vi "serial_load.vi"(5 "new_data_available":bool, 7 "read_buffer_in":string, 8 "data_available_in":T1, 9 "freq_available_in":bool, 10 "s11_data_array_in":dbl[][](array[numeric]), 11 "freq_array_in":dbl[](array[numeric])) -> (0 "data_available_out":T1, 1 "freq_available_out":bool, 2 "data_array_out":dbl[][](array[numeric]), 3 "freq_array_out":dbl[](array[numeric]), 4 "sweep_data":dbl[](array[numeric]), 6 "sweep_data_available":bool)   [LabVIEW 2025]
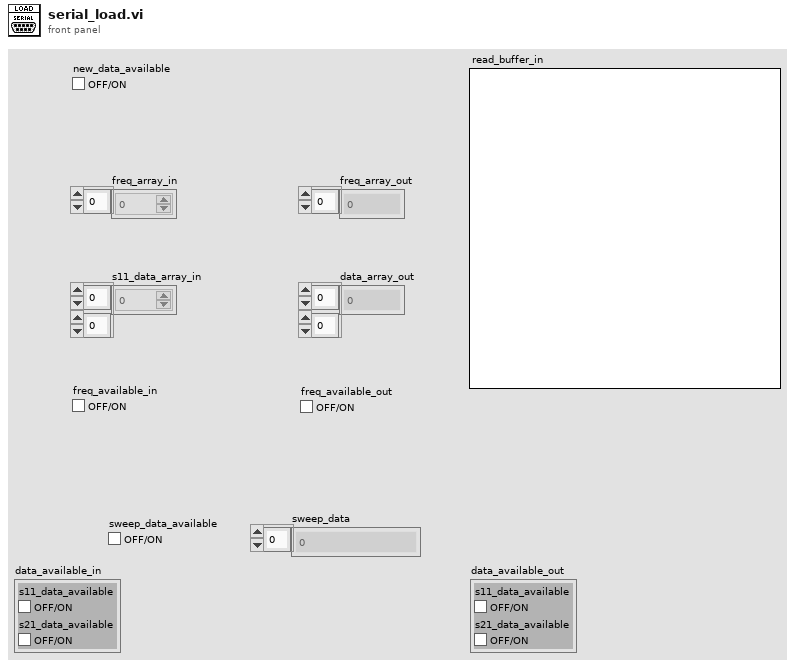
[diagram p1: front panel]
types:
  T1 = cluster{"s11_data_available":bool, "s21_data_available":bool}
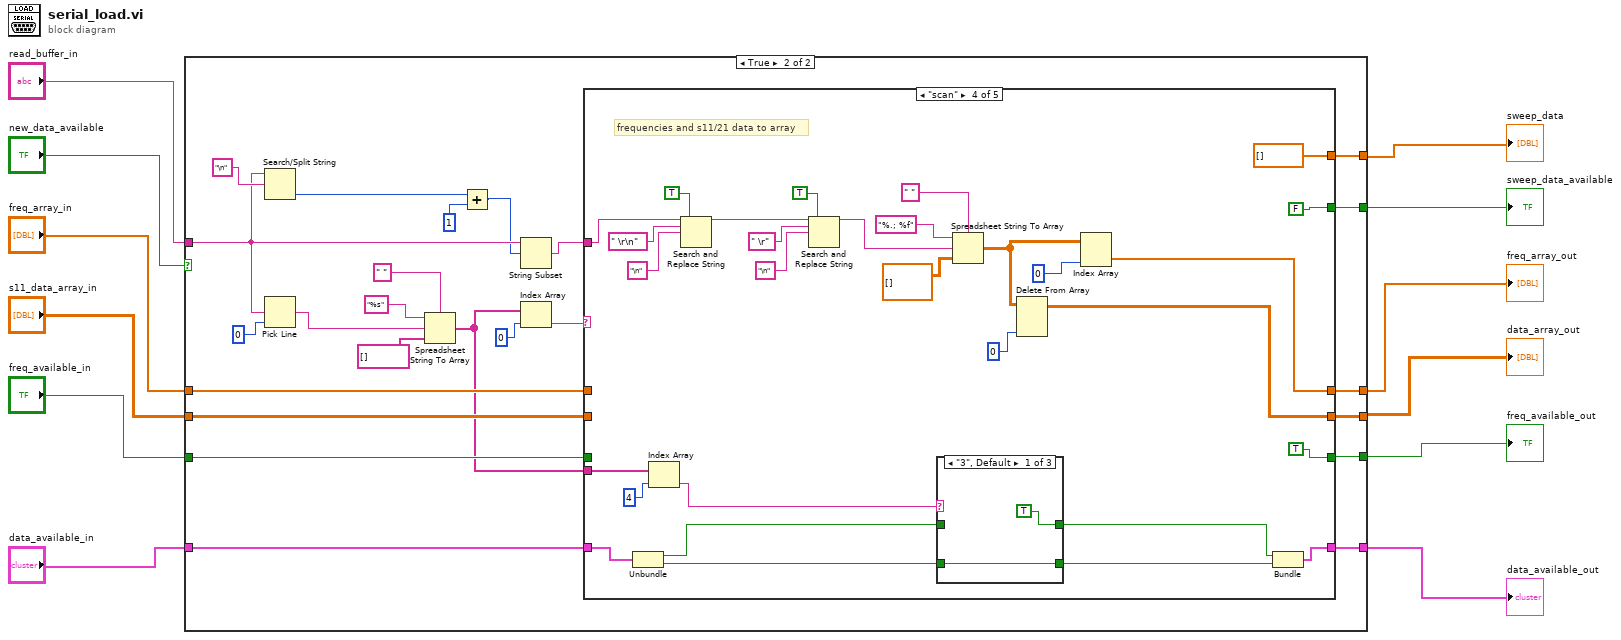
[diagram p0: block diagram]
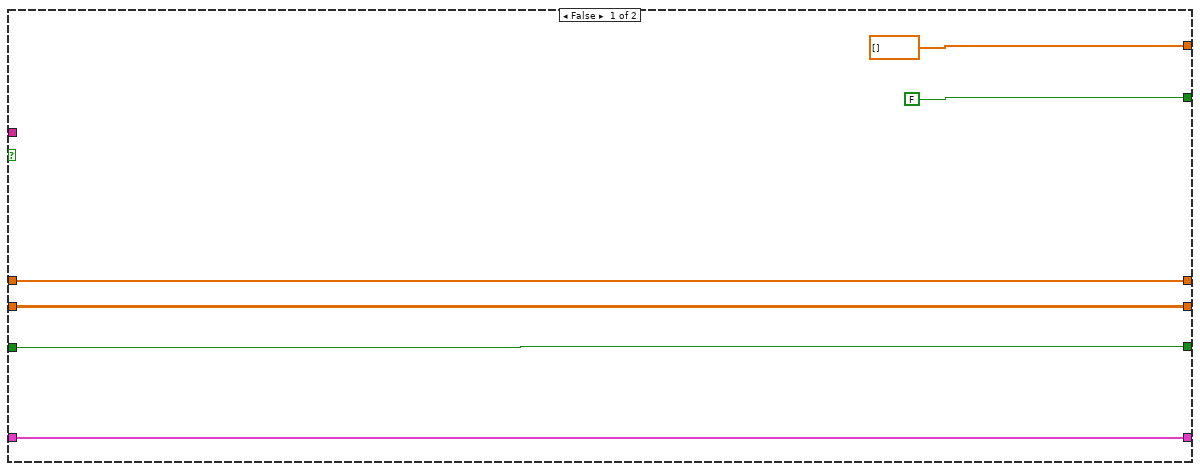
[diagram p2: hidden frame]
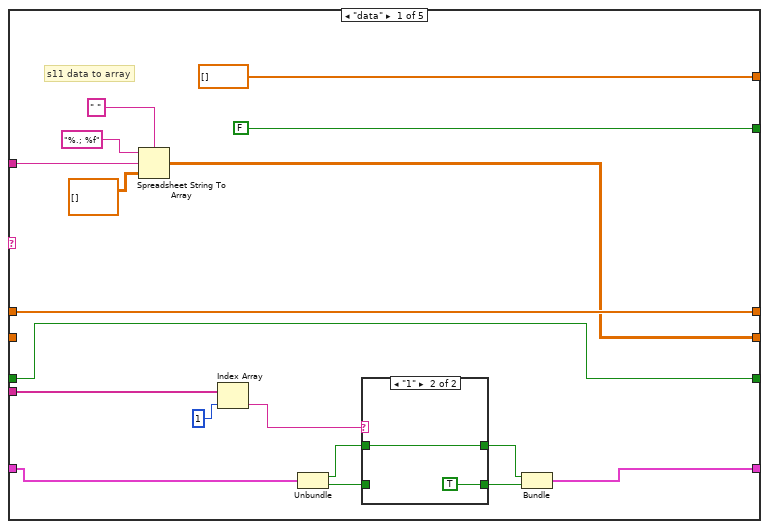
[diagram p3: hidden frame]
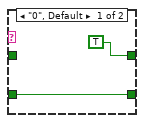
[diagram p4: hidden frame]
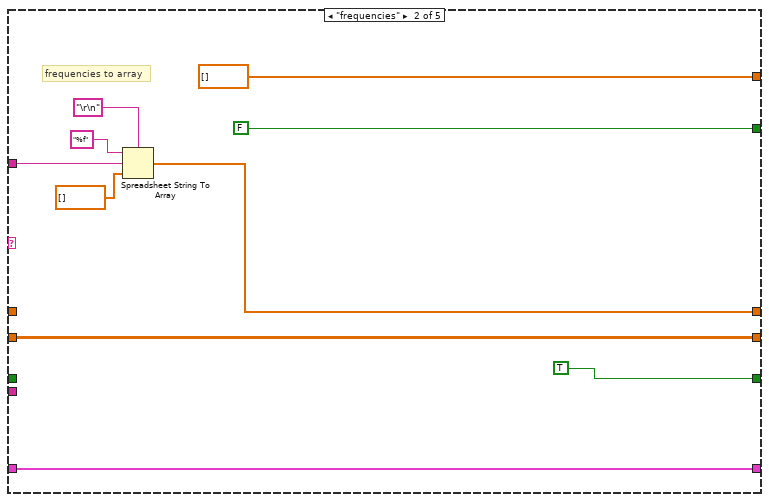
[diagram p5: hidden frame]
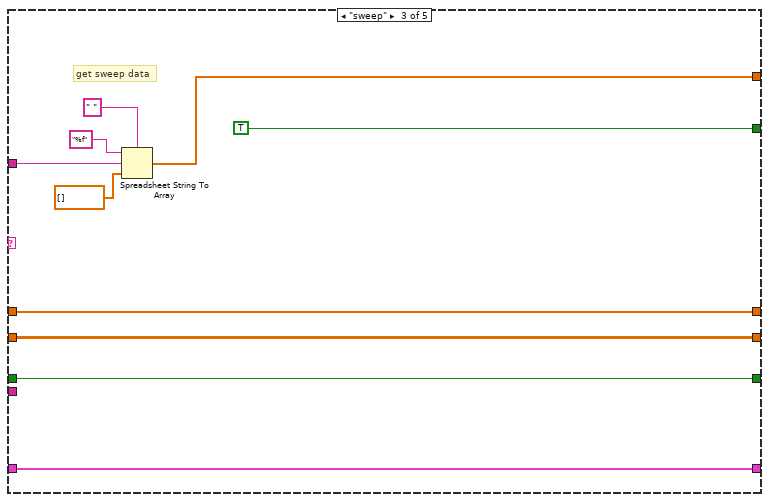
[diagram p6: hidden frame]
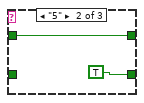
[diagram p7: hidden frame]
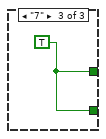
[diagram p8: hidden frame]
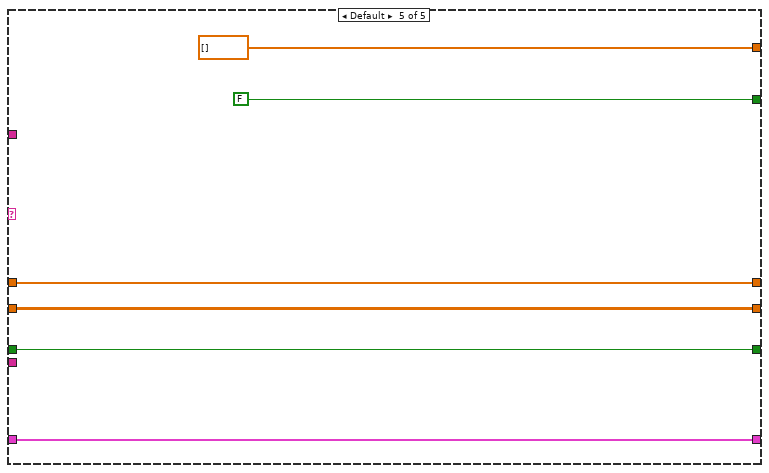
[diagram p9: hidden frame]
diagram:
  n1 = case shown="True" "new_data_available" {
    tunnel: "read_buffer_in" -> [_ w32]
    tunnel: [w18 w31] -> w3
    tunnel: "freq_available_in" -> [w18 w41]
    tunnel: "freq_array_in" -> [w17 w40]
    tunnel: [w17 w39] -> w11
    tunnel: "s11_data_array_in" -> [w16 w38]
    tunnel: [w16 w37] -> w12
    tunnel: [dbl[] [] ("array type (2D Dbl)") w35] -> w5
    tunnel: [FALSE w34] -> w4
    tunnel: [w13 w27] -> w2
    tunnel: "data_available_in" -> [w13 w26]
    frame False {
    }
    frame True {
      n2 = Search/Split String(string=w32, search string/char (-)="\n") -> (offset of match=w30:i32)  [unwired: 1 in, 2 out]
      n3 = Pick Line(multi-line string=w32, line index=0) -> (output string=w22:string)  [unwired: 1 in]
      n4 = Spreadsheet String To Array(delimiter (Tab)=" ", format string="%s", spreadsheet string=w22, array type (2D Dbl)=string[] []) -> (array=w19:string[])
      n5 = Add(x=w30, y=1) -> (x+y=w28:i32)
      n6 = String Subset(string=w32, offset (0)=w28) -> (substring=w33:string)  [unwired: 1 in]
      n7 = Index Array(array=w19, index=0) -> (element=w20:string)
      n8 = case shown="\"scan\"" w20 {
        tunnel: w33 -> [w57 w72 w79 w98 _]
        tunnel: [w46 TRUE w78 TRUE ("freq_available_in") w124] -> w31
        tunnel: w41 -> [w46 _ w78 _ w124]
        tunnel: w40 -> [w56 _ w84 _ w123]
        tunnel: [w56 w66 w84 w107 w123] -> w39
        tunnel: w38 -> [_ w70 w83 _ w122]
        tunnel: [w49 w70 w83 w93 w122] -> w37
        tunnel: [dbl[] [] ("array type (2D Dbl)") dbl[] [] ("array type (2D Dbl)") w76 dbl[] [] ("array type (2D Dbl)") dbl[] [] ("array type (2D Dbl)")] -> w35
        tunnel: [FALSE FALSE TRUE FALSE FALSE] -> w34
        tunnel: [w48 w65 w75 w101 w119] -> w27
        tunnel: w26 -> [w47 w65 w75 w85 w119]
        tunnel: w19 -> [w44 _ _ w94 _]
        frame "data" {
          # "s11 data to array"
          n9 = Spreadsheet String To Array(delimiter (Tab)=" ", format string="%.; %f", spreadsheet string=w57, array type (2D Dbl)=dbl[][] []) -> (array=w49:dbl[][])
          n10 = Index Array(array=w44, index=1) -> (element=w43:string)
          n11 = Unbundle(w47) -> ("s11_data_available"=w51:bool, "s21_data_available"=w50:bool)
          n12 = case shown="\"1\"" w43 {
            tunnel: [w61 TRUE] -> w53
            tunnel: [TRUE w63] -> w52
            tunnel: w51 -> [_ w63]
            tunnel: w50 -> [w61 _]
            frame "0", Default {
            }
            frame "1" {
            }
          }
          n13 = Bundle("s11_data_available"=w52, "s21_data_available"=w53) -> (w48:T1)  [unwired: 1 in]
        }
        frame "frequencies" {
          # "frequencies to array"
          n14 = Spreadsheet String To Array(delimiter (Tab)="\r\n", format string="%f", spreadsheet string=w72, array type (2D Dbl)=dbl[] []) -> (array=w66:dbl[])
        }
        frame "sweep" {
          # "get sweep data"
          n15 = Spreadsheet String To Array(delimiter (Tab)=" ", format string="%f", spreadsheet string=w79, array type (2D Dbl)=dbl[] []) -> (array=w76:dbl[])
        }
        frame "scan" {
          # "frequencies and s11/21 data to array"
          n16 = Unbundle(w85) -> ("s11_data_available"=w103:bool, "s21_data_available"=w102:bool)
          n17 = Index Array(array=w94, index=4) -> (element=w95:string)
          n18 = Search and Replace String(replace all?=TRUE ("replace all? (F)"), input string=w98, search string=" \r\n", replace string="\n" ("replace string (\"\")")) -> (result string=w87:string)  [unwired: 4 in, 3 out]
          n19 = Search and Replace String(replace all?=TRUE ("replace all? (F)"), input string=w87, search string=" \r", replace string="\n" ("replace string (\"\")")) -> (result string=w88:string)  [unwired: 4 in, 3 out]
          n20 = case shown="\"3\", Default" w95 {
            tunnel: [w114 TRUE w118] -> w105
            tunnel: [TRUE w116 w118] -> w104
            tunnel: w103 -> [_ w116 _]
            tunnel: w102 -> [w114 _ _]
            frame "3", Default {
            }
            frame "5" {
            }
            frame "7" {
              w118 = TRUE
            }
          }
          n21 = Spreadsheet String To Array(delimiter (Tab)=" ", format string="%.; %f", spreadsheet string=w88, array type (2D Dbl)=dbl[][] []) -> (array=w86:dbl[][])
          n22 = Delete From Array(array=w86, index (col)=0) -> (array with subset deleted=w93:dbl[][])  [unwired: 2 in, 1 out]
          n23 = Index Array(array=w86, index (col)=0) -> (element=w107:dbl[])  [unwired: 1 in]
          n24 = Bundle("s11_data_available"=w104, "s21_data_available"=w105) -> (w101:T1)  [unwired: 1 in]
        }
        frame Default {
        }
      }
    }
  }
  "freq_available_out" <- w3
  "data_array_out" <- w12
  "freq_array_out" <- w11
  "sweep_data" <- w5
  "sweep_data_available" <- w4
  "data_available_out" <- w2
